vi "IIR 2nd Order Filter Vec.vi"(7 "initialize":bool, 8 "IIR Filter Cluster":T1, 10 "Initial value":dbl[](array[numeric]) format="%0.2f", 11 "x":dbl[](array[numeric]) format="%0.2f") -> (3 "Filtered X":dbl[](array[numeric]) format="%0.2f")   [LabVIEW 2012]
doc: "Filters <B>x</B> using the cascade form of the IIR filter specified by the <B>IIR Filter Cluster</B>."
panel:
  # "If \"Initial Value\" is supplied and not empty, then we reset to that value, instead of the current input."
  # "Note: this is ONLY for second order filters, though it takes the general filter structure.  This is just for efficiency, or more likely a bad idea."
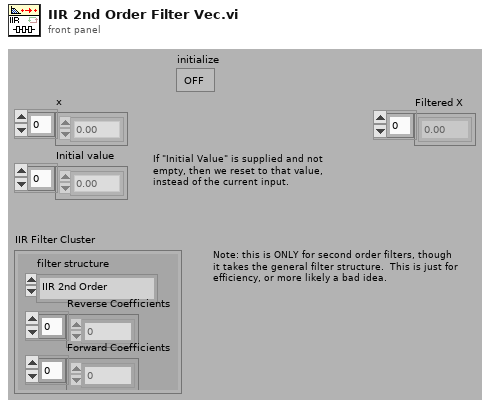
[diagram p1: front panel]
types:
  T1 = cluster{"filter structure":enum32{"IIR 2nd Order", "IIR 4th Order"}, "Reverse Coefficients":dbl[], "Forward Coefficients":dbl[]}
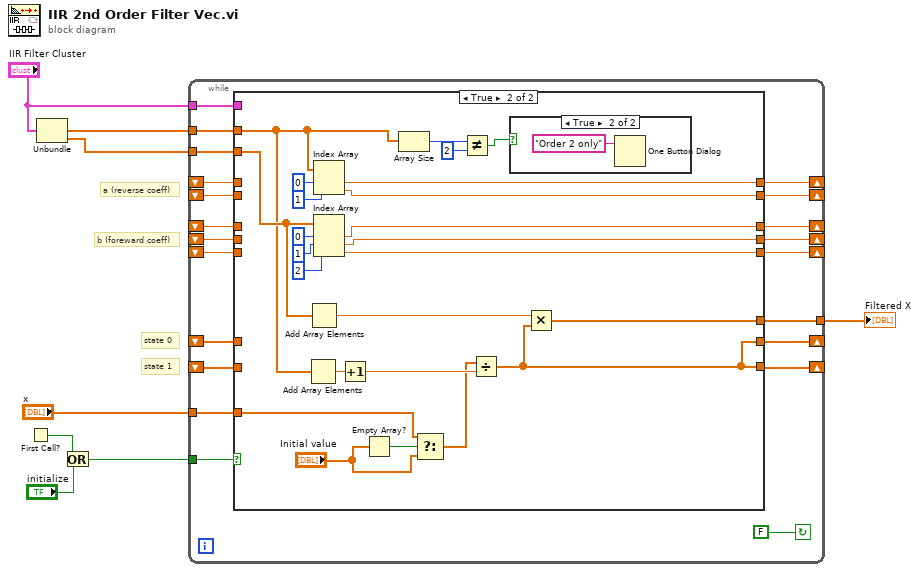
[diagram p0: block diagram]
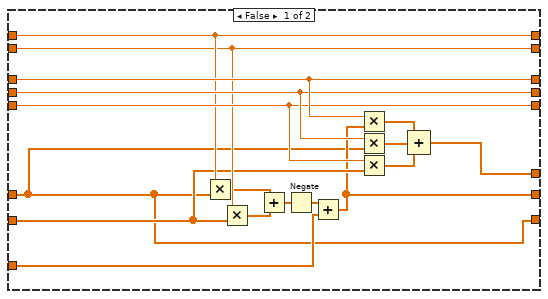
[diagram p2: hidden frame]
diagram:
  # "state 1"
  # "state 0"
  # "b (foreward coeff)"
  # "a (reverse coeff)"
  n1 = First Call?() -> (First Call?: T/F=w6:bool)
  n2 = Unbundle("IIR Filter Cluster") -> ("Reverse Coefficients"=w1:dbl[], "Forward Coefficients"=w2:dbl[])  [unwired: 1 out]
  n3 = Or(x=w6, y="initialize") -> (x .or. y?=w7:bool)
  n4 = while {
    tunnel: "IIR Filter Cluster" -> [w12]
    tunnel: [w15] -> w3
    shift-left: _ -> [w16]
    shift-right: [w14] -> _
    shift-left: _ -> [w17]
    shift-right: [w18] -> _
    shift-left: _ -> [w19]
    shift-right: [w20] -> _
    shift-left: _ -> [w21]
    shift-right: [w22] -> _
    tunnel: "x" -> [w23]
    tunnel: w1 -> [w24]
    shift-left: _ -> [w25]
    shift-right: [w27] -> _
    shift-left: _ -> [w26]
    shift-right: [w28] -> _
    tunnel: w2 -> [w29]
    tunnel: w7 -> [w11]
    shift-right: [w10] -> _
    shift-left: _ -> [w9]
    stop <- FALSE continue-if-true
    n5 = case shown="True" w11 {
      tunnel: w29 -> [_ w60]
      tunnel: [w45 w62] -> w28
      tunnel: [w44 w61] -> w27
      tunnel: w26 -> [w45 _]
      tunnel: w25 -> [w44 _]
      tunnel: w24 -> [_ w49]
      tunnel: w23 -> [w40 w52]
      tunnel: [w42 w67] -> w22
      tunnel: w21 -> [w42 _]
      tunnel: [w46 w63] -> w20
      tunnel: w19 -> [w46 _]
      tunnel: [w43 w68] -> w18
      tunnel: w17 -> [w43 _]
      tunnel: [w41 w55] -> w15
      tunnel: w16 -> [w30 _]
      tunnel: [w31 w57] -> w14
      tunnel: w12 -> [_ _]
      tunnel: [w30 w57] -> w10
      tunnel: w9 -> [w32 _]
      frame False {
        n6 = Multiply(x=w43, y=w30) -> (x*y=w39:dbl[])
        n7 = Multiply(x=w42, y=w32) -> (x*y=w38:dbl[])
        n8 = Add(x=w39, y=w38) -> (x+y=w37:dbl[])
        n9 = Negate(x=w37) -> (-x=w36:dbl[])
        n10 = Add(x=w36, y=w40) -> (x+y=w31:dbl[])
        n11 = Multiply(x=w46, y=w31) -> (x*y=w35:dbl[])
        n12 = Multiply(x=w45, y=w30) -> (x*y=w34:dbl[])
        n13 = Multiply(x=w44, y=w32) -> (x*y=w33:dbl[])
        n14 = Compound Arithmetic op=ADD(w35, w34, w33) -> (w41:dbl[])
      }
      frame True {
        n15 = Add Array Elements(numeric array=w49) -> (sum=w59:dbl)
        n16 = Add Array Elements(numeric array=w60) -> (sum=w56:dbl)
        n17 = Index Array(array=w49, index #1=0 ("index"), index #2=1 ("index")) -> (element #1=w68:dbl, element #2=w67:dbl)
        n18 = Index Array(array=w60, index #1=0 ("index"), index #2=1 ("index"), index #3=2 ("index")) -> (element #1=w63:dbl, element #2=w62:dbl, element #3=w61:dbl)
        n19 = Increment(x=w59) -> (x+1=w58:dbl)
        n20 = Empty Array?(array="Initial value") -> (empty?=w54:bool)
        n21 = Array Size(array=w49) -> (size(s)=w50:i32)
        n22 = Select(t=w52, s=w54, f="Initial value") -> (s? t:f=w51:dbl[])
        n23 = Not Equal?(x=w50, y=2) -> (x != y?=w47:bool)
        n24 = Divide(x=w51, y=w58) -> (x/y=w57:dbl[])
        n25 = case shown="True" w47 {
          frame False {
          }
          frame True {
            n26 = One Button Dialog(message="Order 2 only") -> ()  [unwired: 1 in, 1 out]
          }
        }
        n27 = Multiply(x=w56, y=w57) -> (x*y=w55:dbl[])
      }
    }
  }
  "Filtered X" <- w3
